vi "scale-name-sorter.vi"(11 "Cluster":T1) -> (3 "Array":string[][](array[string]))   [LabVIEW 2019]
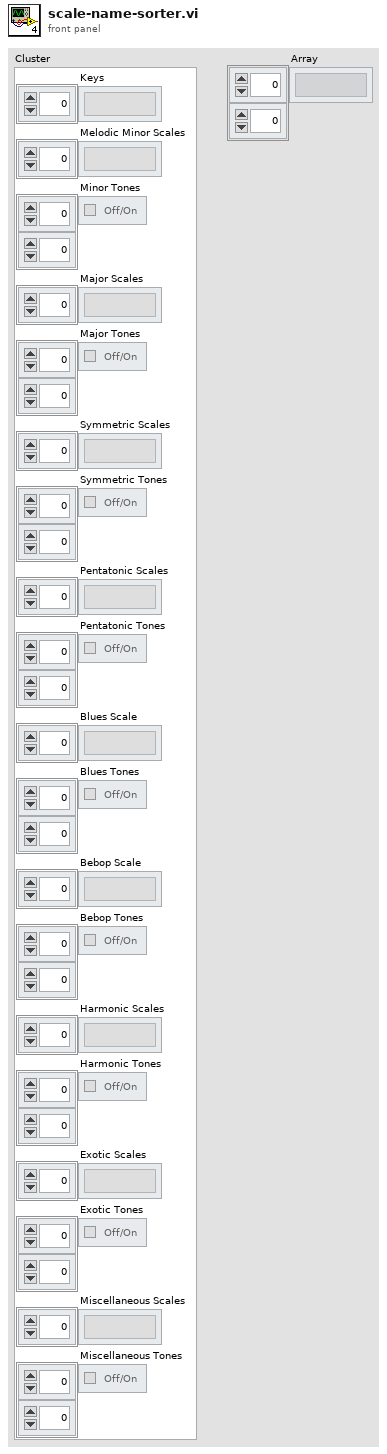
[diagram p1: front panel]
types:
  T1 = cluster{"Keys":string[], "Melodic Minor Scales":string[], "Minor Tones":bool[][], "Major Scales":string[], "Major Tones":bool[][], "Symmetric Scales":string[], "Symmetric Tones":bool[][], "Pentatonic Scales":string[], "Pentatonic Tones":bool[][], "Blues Scale":string[], "Blues Tones":bool[][], "Bebop Scale":string[], "Bebop Tones":bool[][], "Harmonic Scales":string[], "Harmonic Tones":bool[][], "Exotic Scales":string[], "Exotic Tones":bool[][], "Miscellaneous Scales":string[], "Miscellaneous Tones":bool[][]}
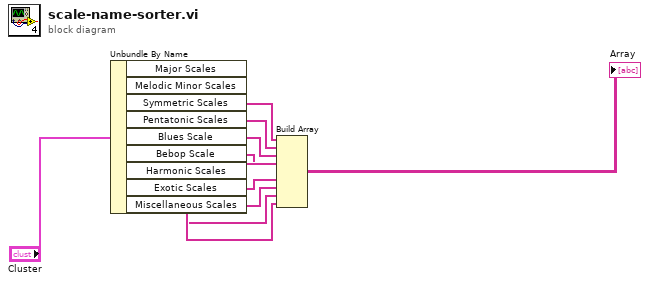
[diagram p0: block diagram]
diagram:
  n1 = Unbundle By Name("Cluster") -> ("Major Scales"=w1:string[], "Melodic Minor Scales"=w2:string[], "Symmetric Scales"=w3:string[], "Pentatonic Scales"=w4:string[], "Blues Scale"=w5:string[], "Bebop Scale"=w6:string[], "Harmonic Scales"=w7:string[], "Exotic Scales"=w8:string[], "Miscellaneous Scales"=w9:string[])
  n2 = Build Array(w1, w2, w3, w4, w5, w6, w7, w8, w9) -> (→"Array":string[][])
